vi "CreatePrivateEvents.vi"(8 "error in (no error)":errorcluster, 11 "XYStage":refnum<class "XYStage.lvclass">) -> (0 "error out":errorcluster, 3 "XYStage out":refnum<class "XYStage.lvclass">)   [LabVIEW 2013, in "XYStage.lvclass"]
doc: "---------------------------------------------------------------\nJKI State Machine Objects™\nhttp://jki.net/state-machine-objects/\nCopyright (C) 2005-2015, JKI <info@jki.net>\nALL RIGHTS RESERVEDJKI State Machine Objects (SMO) 1.0.0.4\nJKI - JKI\nCopyright (c) 2015, JKI"
uses:
  XYStage.lvclass
  <vilib>/JKI/JKI SMO/SMO/SMO.lvclass
  Typedefs/(real)Coords--Cluster.ctl
  Typedefs/PrivateEvents--XYStage.MoveToNamedPosition.ctl
  Typedefs/PrivateEvents--XYStage.StorePosition.ctl
  Typedefs/PrivateEvents--XYStage.Home.ctl
panel:
  # "For instructions on how to use the JKI State Machine Objects, examples and video tutorials, visit:\nhttp://jki.net/state-machine-objects/\n\nJKI State Machine Objects™\nhttp://jki.net/state-machine-objects/\nCopyright (C) 2005-2015, JKI <info@jki.net>\nALL RIGHTS RESERVED"
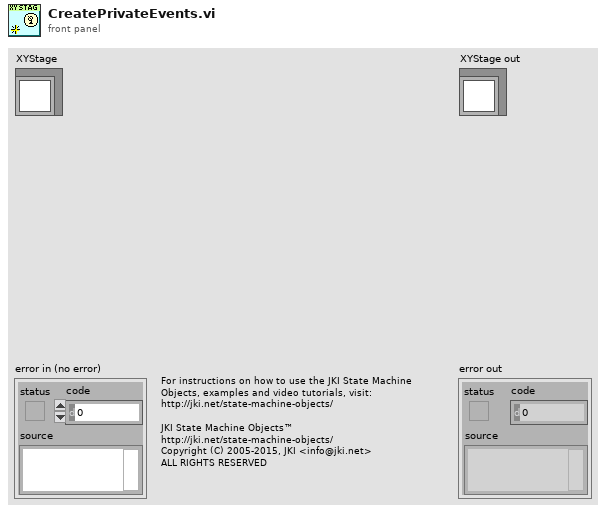
[diagram p1: front panel]
types:
  T1 = typedef "XYStage.lvclass/PrivateData--Ref.ctl" = refnum<data-value>
  T2 = typedef "XYStage.lvclass/PrivateEvents--XYStage.Home.ctl" = bool
  T3 = typedef "XYStage.lvclass/PrivateEvents--XYStage.StorePosition.ctl" = cluster{"Name":string, "Coords":T4}
  T4 = typedef "XYStage.lvclass/(real)Coords--Cluster.ctl" = cluster{"X":dbl, "Y":dbl}
  T5 = typedef "XYStage.lvclass/PrivateEvents--XYStage.MoveToNamedPosition.ctl" = string
  T6 = typedef "XYStage.lvclass/PrivateData--Cluster.ctl" = cluster{"Dependencies":T7, "Public Events":T8, "Protected Events":T9, "Private Events":T10, "Configuration":T11, "Target":T12, "Move Parameters":T14}
  T7 = typedef "XYStage.lvclass/Dependencies--Cluster.ctl" = cluster{"Positions":refnum<class "SMO.Dictionary.Variant.lvclass">}
  T8 = typedef "XYStage.lvclass/PublicEvents--Cluster.ctl" = cluster{"MoveComplete":refnum<user-event>, "NewPosition":refnum<user-event>, "UpdatedNamedPosition":refnum<user-event>, "MoveStarted":refnum<user-event>}
  T9 = typedef "XYStage.lvclass/ProtectedEvents--Cluster.ctl" = cluster{"API_Template":refnum<user-event>}
  T10 = typedef "XYStage.lvclass/PrivateEvents--Cluster.ctl" = cluster{"MoveAbsolute":refnum<user-event>, "MoveRelative":refnum<user-event>, "MoveToNamedPosition":refnum<user-event>, "StorePosition":refnum<user-event>, "Home":refnum<user-event>}
  T11 = typedef "XYStage.lvclass/Configuration--Cluster.ctl" = cluster{"Real-World Units":string, "Counts per Unit":dbl}
  T12 = typedef "XYStage.lvclass/TargetPositions--Cluster.ctl" = cluster{"Coords":T4, "Counts":T13}
  T13 = typedef "XYStage.lvclass/(counts)Coords--Cluster.ctl" = cluster{"X":i32, "Y":i32}
  T14 = typedef "XYStage.lvclass/MoveParameters--Cluster.ctl" = cluster{"Velocity (units/s)":dbl, "Acceleration (units/s^2)":dbl}
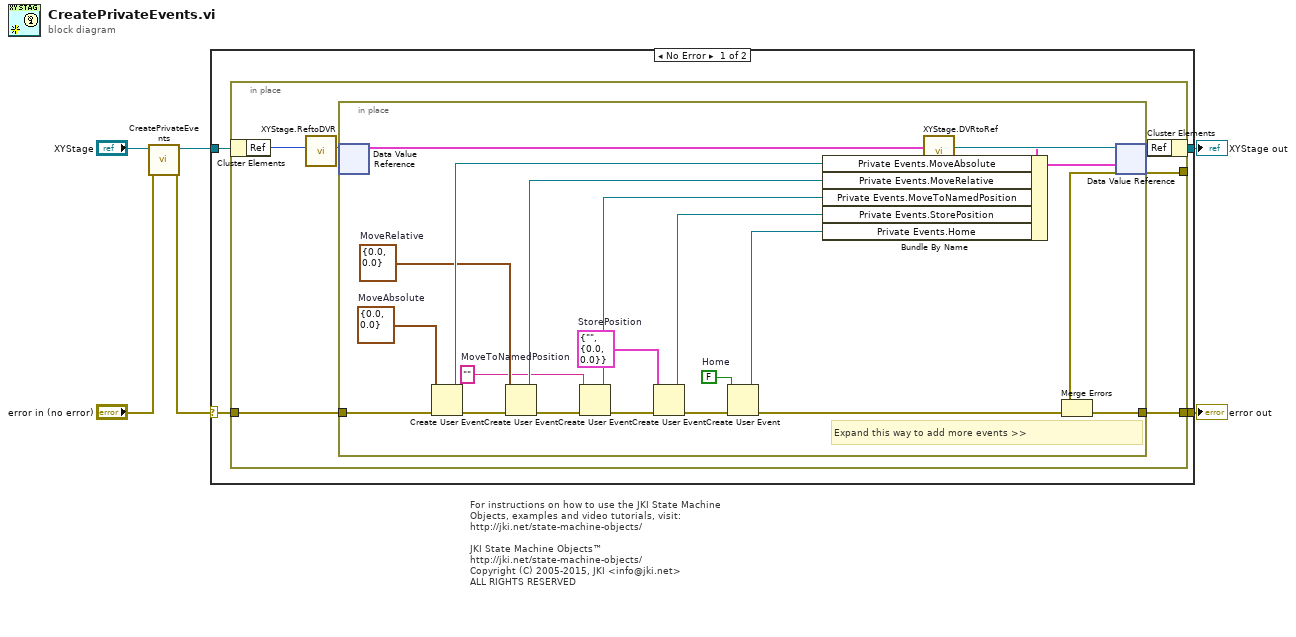
[diagram p0: block diagram]
diagram:
  # "For instructions on how to use the JKI State Machine Objects, examples and video tutorials, visit:\nhttp://jki.net/state-machine-objects/\n\nJKI State Machine Objects™\nhttp://jki.net/state-machine-objects/\nCopyright (C) 2005-2015, JKI <info@jki.net>\nALL RIGHTS RESERVED"
  n1 = call-parent "CreatePrivateEvents.vi"("error in (no error)"="error in (no error)", "SMO"="XYStage") -> ("error out"=w1:errorcluster, "SMO out"=w3:refnum<class "XYStage.lvclass">)  [unwired: 8 in]
  n2 = case shown="No Error" w1 {
    selector: w1 -> [w10 w39]
    tunnel: [w8 w39] -> w5
    tunnel: [w11 w38] -> w6
    tunnel: w3 -> [w12 w38]
    frame No Error {
      n3 = in-place {
        in-place-border: w10 -> [w19]
        in-place-border: [w16] -> w7
        in-place-border: [w15] -> w9
        n4 = in-place-cluster #1(w12) -> ("Ref"=w18:u32)
        n5 = call "XYStage.ReftoDVR.vi"("Ref"=w18) -> ("Ref"=w14:T1)  [unwired: 10 in]
        n6 = in-place {
          in-place-border: w19 -> [w37]
          in-place-border: [w23] -> w16
          w22 = T2 FALSE  # Home
          w25 = T3 {"Name"="", "Coords"={"X"=0.0, "Y"=0.0}}  # StorePosition
          w28 = T5 ""  # MoveToNamedPosition
          w30 = T4 {"X"=0.0, "Y"=0.0}  # MoveRelative
          w31 = T4 {"X"=0.0, "Y"=0.0}  # MoveAbsolute
          # "Expand this way to add more events >>"
          n7 = in-place-dvr #2(w14) -> (w20:T6)  [unwired: 1 out]
          n8 = Create User Event(user event datatype=w31, error in=w37) -> (user event=w34:refnum<user-event>, error out=w35:errorcluster)
          n9 = Create User Event(user event datatype=w30, error in=w35) -> (user event=w32:refnum<user-event>, error out=w33:errorcluster)
          n10 = Create User Event(user event datatype=w28, error in=w33) -> (user event=w27:refnum<user-event>, error out=w29:errorcluster)
          n11 = Create User Event(user event datatype=w25, error in=w29) -> (user event=w24:refnum<user-event>, error out=w26:errorcluster)
          n12 = Create User Event(user event datatype=w22, error in=w26) -> (user event=w21:refnum<user-event>, error out=w23:errorcluster)
          n13 = Bundle By Name(cluster=w20, "Private Events.MoveAbsolute"=w34, "Private Events.MoveRelative"=w32, "Private Events.MoveToNamedPosition"=w27, "Private Events.StorePosition"=w24, "Private Events.Home"=w21) -> (w36:T6)
          n14 = in-place-dvr #2(w36) -> (w17:T1, w15:errorcluster)
        }
        n15 = call "XYStage.DVRtoRef.vi"("Ref"=w17) -> ("Ref"=w13:u32)  [unwired: 10 in]
        n16 = in-place-cluster #1("Ref"=w13) -> (w11:refnum<class "XYStage.lvclass">)
      }
      n17 = Merge Errors(w9, w7) -> (w8:errorcluster)
    }
    frame Error {
    }
  }
  "error out" <- w5
  "XYStage out" <- w6
